vi "Tables.vi"(8 "1D Array":u64[](array[numeric]), 10 "Dimension":i64, 11 "2D Array":u64[][](array[numeric])) -> (0 "1D Table Control 2":string[][](table), 3 "2D Table Control":string[][](table))   [LabVIEW 2023]
panel:
  out "Out":string[][](array[string])
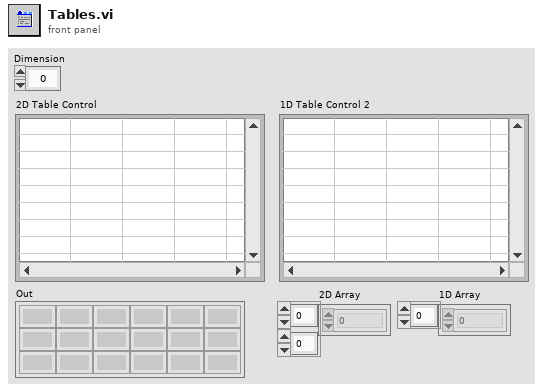
[diagram p1: front panel]
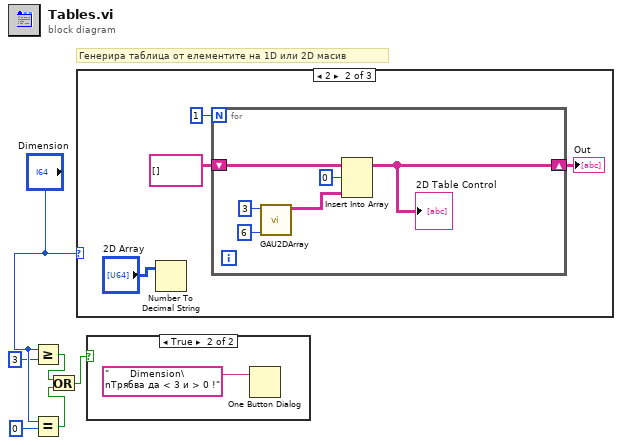
[diagram p0: block diagram]
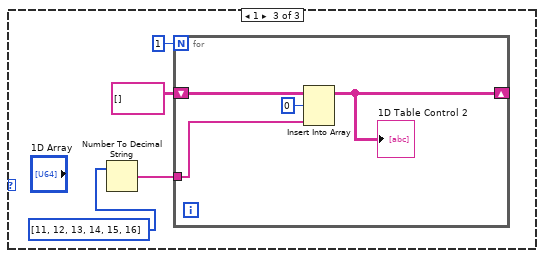
[diagram p4: hidden frame]
diagram:
  # "Генерира таблица от елементите на 1D или 2D масив"
  n1 = Greater Or Equal?(x="Dimension", y=i64 3) -> (x >= y?=w2:bool)
  n2 = Equal?(x="Dimension", y=i64 0) -> (x = y?=w3:bool)
  n3 = Or(x=w2, y=w3) -> (x .or. y?=w1:bool)
  n4 = case shown="2" "Dimension" {
    frame 0, Default {
    }
    frame 2 {
      n5 = Number To Decimal String(number="2D Array") -> ()  [unwired: 1 in, 1 out]
      n6 = for {
        N: 1 -> [_]
        shift-right: [w11] -> w7
        shift-left: string[][] [] -> [w16]
        n7 = call "GAU2DArray.vi"("Colums"=6, "Rows"=3) -> ("2D String Array"=w12:string[][])  [unwired: 8 in, 1 out]
        n8 = Insert Into Array "Insert Into Array"(array=w16, index (row)=0 ("index"), new element=w12) -> (w11:string[][])  [unwired: 1 in]
        "2D Table Control" <- w11
      }
      "Out" <- w7
    }
    frame 1 {
      n9 = Number To Decimal String(number=i32[] [11, 12, 13, 14, 15, 16]) -> (decimal integer string=w19:string[])  [unwired: 1 in]
      n10 = for {
        N: 1 -> [_]
        shift-right: [w22] -> _
        shift-left: string[][] [] -> [w24]
        tunnel: w19 -> [w21]
        n11 = Insert Into Array "Insert Into Array"(array=w24, index (row)=0 ("index"), new element=w21) -> (w22:string[][])  [unwired: 1 in]
        "1D Table Control 2" <- w22
      }
    }
  }
  n12 = case shown="True" w1 {
    frame False {
    }
    frame True {
      n13 = One Button Dialog(message="       Dimension\nТрябва да < 3 и > 0 !") -> ()  [unwired: 1 in, 1 out]
    }
  }
